vi "Unit Test.vi"() -> ()   [LabVIEW 2018]
uses:
  PPLs/DMM/Parent/DMM.lvlibp/Custom Controls/Measurement Type.ctl
  PPLs/DMM/Parent/DMM.lvlibp/DMM.lvclass
panel:
  in  "OK Button":bool
  in  "Resolution":dbl
  in  "Range":dbl
  in  "AutoRange?":bool
  out "Value":dbl
  out "Model":string
  out "Serial Number":string
  out "Firmware":string
  out "error out":errorcluster
  in  "error in (no error)":errorcluster
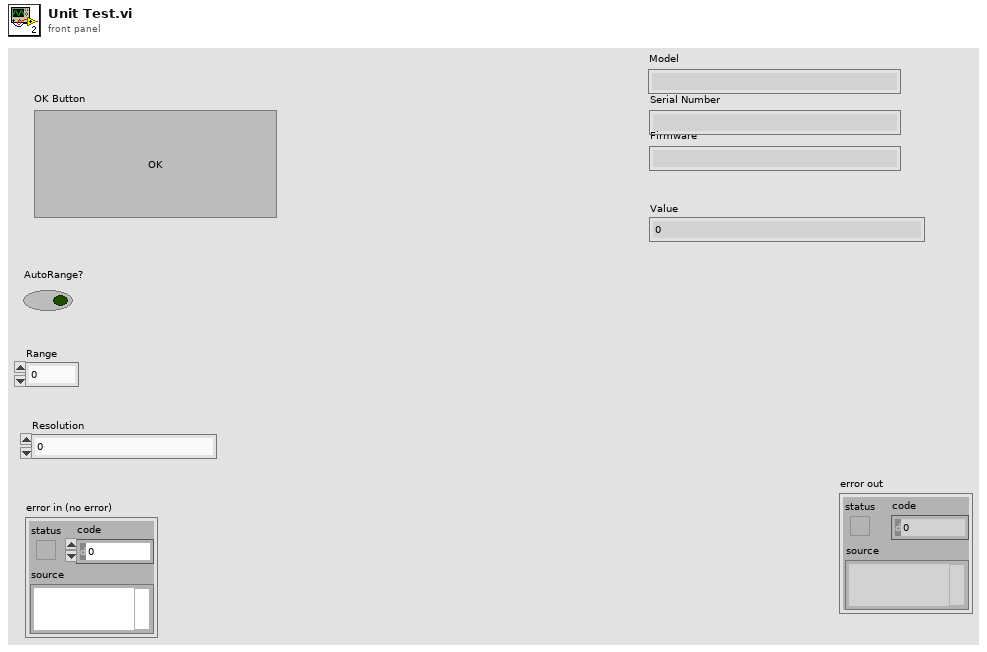
[diagram p1: front panel]
types:
  T1 = typedef "DMM.lvlibp/DMM.lvclass/Measurement Type.ctl" = u32
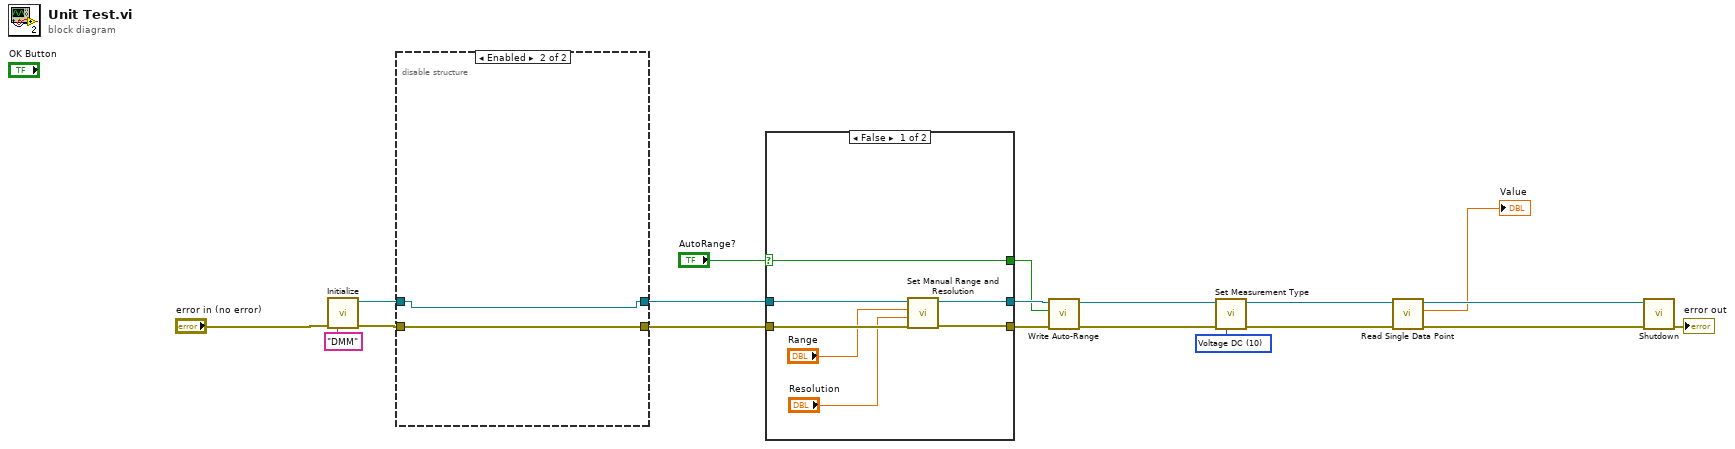
[diagram p0: block diagram]
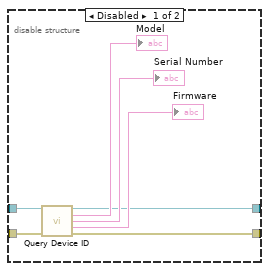
[diagram p2: hidden frame]
diagram:
  w10 = T1 10 items=["Continuity", "Current AC", "Current DC", "Diode", "Frequency", "Resistance 4-wire", "Period", "Resistance 2-wire", "Temperature", "Voltage AC", "Voltage DC", "Voltage DC Ratio", "Capacitance"] ("Measurement Type")
  n1 = call "Initialize.vi"("error in (no error)"="error in (no error)", "Device"="DMM") -> ("error out"=w13:errorcluster, "DMM out"=w14:refnum<class "DMM.lvclass">)  [unwired: 8 in]
  n2 = disable-structure shown="Enabled" {
    disable-tunnel: w14 -> [w26 w28]
    disable-tunnel: w13 -> [w25 w27]
    disable-tunnel: [w21 w27] -> w5
    disable-tunnel: [w20 w28] -> w3
    frame Disabled {
      n3 = call-dynamic "Query Device ID.vi"("DMM in"=w26, "error in (no error)"=w25) -> ("DMM out"=w20:refnum<class "DMM.lvclass">, "Model"=→"Model":string, "Serial Number"=→"Serial Number":string, "Firmware"=→"Firmware":string, "error out"=w21:errorcluster)  [unwired: 9 in]
    }
    frame Enabled {
    }
  }
  n4 = case shown="False" "AutoRange?" {
    selector: "AutoRange?" -> [w35 w36]
    tunnel: [w31 w38] -> w6
    tunnel: w5 -> [w32 w38]
    tunnel: [w33 w37] -> w4
    tunnel: w3 -> [w34 w37]
    tunnel: [w35 w36] -> w1
    frame False {
      n5 = call-dynamic "Set Manual Range and Resolution.vi"("error in (no error)"=w32, "Resolution"="Resolution", "Range"="Range", "DMM in"=w34) -> ("error out"=w31:errorcluster, "DMM out"=w33:refnum<class "DMM.lvclass">)  [unwired: 6 in]
    }
    frame True {
    }
  }
  n6 = call "Write Auto-Range.vi"("error in (no error)"=w6, "Auto-Range"=w1, "DMM in"=w4) -> ("error out"=w8:errorcluster, "DMM out"=w7:refnum<class "DMM.lvclass">)  [unwired: 7 in]
  n7 = call-dynamic "Set Measurement Type.vi"("error in (no error)"=w8, "Measurement Type"=w10, "DMM in"=w7) -> ("error out"=w11:errorcluster, "DMM out"=w12:refnum<class "DMM.lvclass">)  [unwired: 7 in]
  n8 = call-dynamic "Read Single Data Point.vi"("error in (no error)"=w11, "DMM in"=w12) -> ("error out"=w17:errorcluster, "Value"=→"Value":dbl, "DMM out"=w16:refnum<class "DMM.lvclass">)  [unwired: 7 in]
  n9 = call "Shutdown.vi"("error in (no error)"=w17, "DMM in"=w16) -> ("error out"=→"error out":errorcluster)  [unwired: 8 in, 1 out]
